vi "Timing FGV.vi"(8 "error in (no error)":errorcluster, 9 "Target time (s)":dbl format="%#_13g", 10 "Index":i32, 11 "Method (Get Time)":enum16{"Start", "Stop", "Reset", "Get Time"}(ring)=enum."Get Time") -> (0 "error out":errorcluster, 2 "Done":bool, 3 "Time Remaining(s)":dbl)   [LabVIEW 2014, in "Timing and Stabilization.lvlib"]
uses:
  Timing and Stabilization.lvlib
panel:
  out "Running":bool
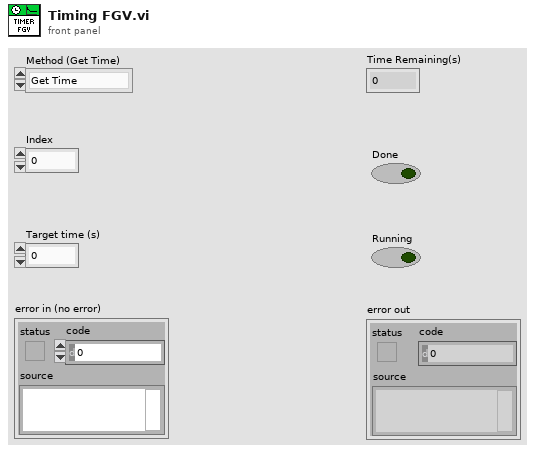
[diagram p1: front panel]
types:
  T1 = cluster{"Start Time":dbl, "Time Remaining":dbl, "Running":bool, "Done":bool}
  T2 = cluster{"Start Time":dbl, "Time Remaining":dbl, "Running":bool, "Done":bool}[]
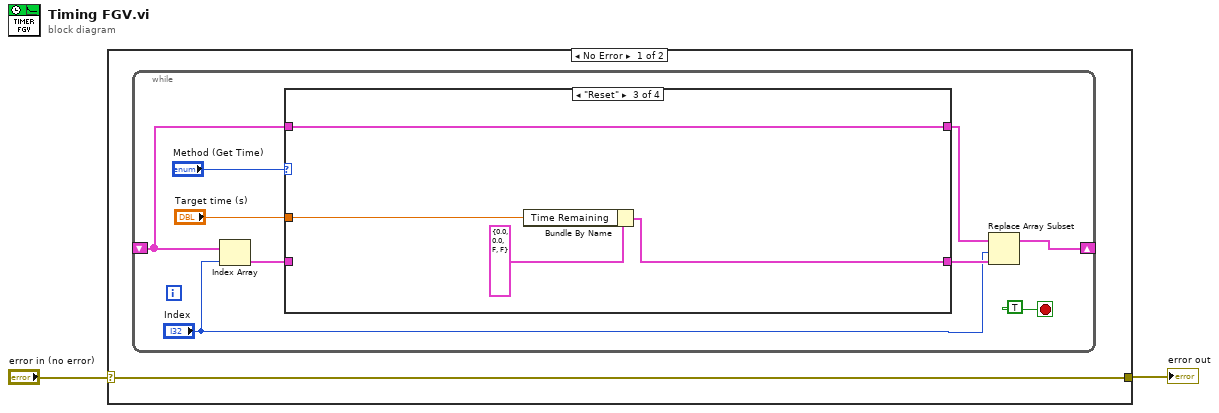
[diagram p0: block diagram]
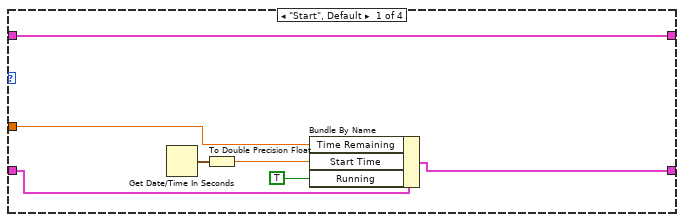
[diagram p2: hidden frame]
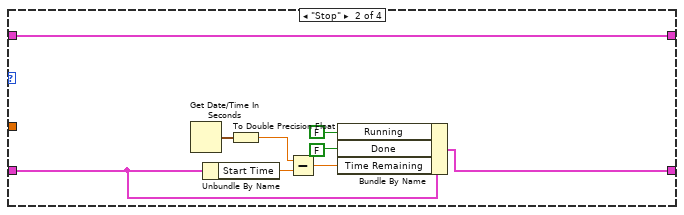
[diagram p3: hidden frame]
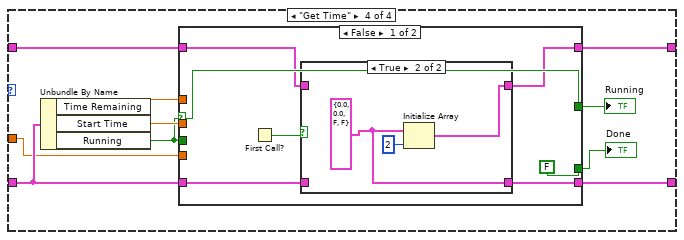
[diagram p4: hidden frame]
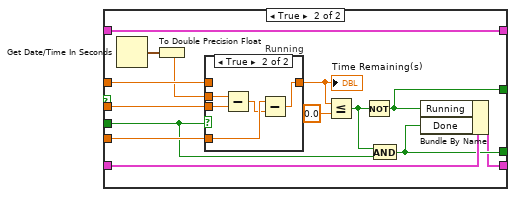
[diagram p6: hidden frame]
diagram:
  n1 = case shown="No Error" "error in (no error)" {
    selector: "error in (no error)" -> [w3 w75]
    tunnel: [w3 w75] -> w1
    frame No Error {
      n2 = while {
        shift-right: [w9] -> _
        shift-left: _ -> [w5]
        stop <- TRUE stop-if-true
        n3 = Index Array(array=w5, index="Index") -> (element=w7:T1)
        n4 = case shown="\"Reset\"" "Method (Get Time)" {
          tunnel: [w13 w22 w30 w37] -> w10
          tunnel: w7 -> [w18 w26 _ w40]
          tunnel: "Target time (s)" -> [w16 _ w31 w39]
          tunnel: w5 -> [w14 w23 w29 w34]
          tunnel: [w14 w23 w29 w33] -> w4
          frame "Start", Default {
            n5 = Get Date/Time In Seconds() -> (seconds since 1Jan1904=w17:timestamp)
            n6 = To Double Precision Float(number=w17) -> (double precision float=w15:dbl)
            n7 = Bundle By Name(cluster=w18, "Time Remaining"=w16, "Start Time"=w15, "Running"=TRUE) -> (w13:T1)
          }
          frame "Stop" {
            n8 = Get Date/Time In Seconds() -> (seconds since 1Jan1904=w25:timestamp)
            n9 = Unbundle By Name(w26) -> ("Start Time"=w27:dbl)
            n10 = To Double Precision Float(number=w25) -> (double precision float=w24:dbl)
            n11 = Subtract(x=w24, y=w27) -> (x-y=w28:dbl)
            n12 = Bundle By Name(cluster=w26, "Running"=FALSE ("Done"), "Done"=FALSE, "Time Remaining"=w28) -> (w22:T1)
          }
          frame "Reset" {
            n13 = Bundle By Name(cluster=T1 {"Start Time"=0.0, "Time Remaining"=0.0, "Running"=FALSE, "Done"=FALSE}, "Time Remaining"=w31) -> (w30:T1)
          }
          frame "Get Time" {
            n14 = Unbundle By Name(w40) -> ("Time Remaining"=w42:dbl, "Start Time"=w41:dbl, "Running"=w36:bool)
            n15 = case shown="False" w36 {
              selector: w36 -> [w48 _]
              tunnel: w42 -> [_ w68]
              tunnel: w41 -> [_ w67]
              tunnel: w40 -> [w46 w64]
              tunnel: w39 -> [_ w63]
              tunnel: [FALSE w61] -> w38
              tunnel: [w45 w58] -> w37
              tunnel: w36 -> [_ w57]
              tunnel: [w48 w56] -> w35
              tunnel: w34 -> [w44 w55]
              tunnel: [w43 w55] -> w33
              frame False {
                n16 = First Call?() -> (First Call?: T/F=w47:bool)
                n17 = case shown="True" w47 {
                  tunnel: w46 -> [w51 _]
                  tunnel: [w51 w52] -> w45
                  tunnel: w44 -> [w50 _]
                  tunnel: [w50 w53] -> w43
                  frame False {
                  }
                  frame True {
                    w52 = T1 {"Start Time"=0.0, "Time Remaining"=0.0, "Running"=FALSE, "Done"=FALSE}
                    n18 = Initialize Array(w52, 2 ("dimension size")) -> (w53:T2)
                  }
                }
              }
              frame True {
                n19 = Get Date/Time In Seconds() -> (seconds since 1Jan1904=w66:timestamp)
                n20 = To Double Precision Float(number=w66) -> (double precision float=w65:dbl)
                n21 = case "Running" shown="True" w57 {
                  tunnel: w65 -> [_ w74]
                  tunnel: w67 -> [_ w73]
                  tunnel: [w69 w72] -> w60
                  tunnel: w68 -> [w69 _]
                  tunnel: w63 -> [_ w71]
                  frame False {
                  }
                  frame True {
                    n22 = Subtract(x=w74, y=w73) -> (x-y=w70:dbl)
                    n23 = Subtract(x=w71, y=w70) -> (x-y=w72:dbl)
                  }
                }
                "Time Remaining(s)" <- w60
                n24 = Less Or Equal?(x=w60, y=0.0) -> (x <= y?=w62:bool)
                n25 = Not(x=w62) -> (.not. x?=w56:bool)
                n26 = And(x=w62, y=w57) -> (x .and. y?=w61:bool)
                n27 = Bundle By Name(cluster=w64, "Running"=w56, "Done"=w61) -> (w58:T1)
              }
            }
            "Running" <- w35
            "Done" <- w38
          }
        }
        n28 = Replace Array Subset(array=w4, new element=w10, index="Index") -> (w9:T2)
      }
    }
    frame Error {
    }
  }
  "error out" <- w1
